vi "LimelightVariables.vi"() -> ()   [LabVIEW 2020]
panel:
  out "Distance":dbl
  out "LedState":dbl
  out "Area":dbl
  out "CamMode":dbl
  out "offsetAngleX":dbl
  out "offsetAngleY":dbl
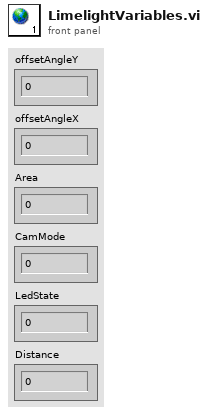
[diagram p1: front panel]
diagram:
